vi "readFromXML.vi"(8 "error in (no error)":errorcluster, 10 "XML in":string, 11 "RotOffset in":refnum<class "RotOffset.lvclass">) -> (0 "error out":errorcluster, 3 "RotOffset out":refnum<class "RotOffset.lvclass">)   [LabVIEW 2022 SP3, in "TCSDataDefinitions.lvlib" / "TCSCommand.lvlib" / "OffsetCommands.lvlib" / "RotOffset.lvclass"]
uses:
  RotOffset.lvclass
  <userlib>/Common/UnitsAndXML/FlattenItemWithUnitToXML/FlattenPlaneAngleToXML/PlaneAngleUnit.ctl
  RotOffset.lvclass/RotOffset.ctl
  RotatorOffsetCommands/RotatorOffsetCommands.lvclass
  <userlib>/Common/UnitsAndXML/UnitsAndXML.lvlib
  <userlib>/Common/XML/XMLParser/XMLParser.lvclass
panel:
  out "iaa":dbl[unit]
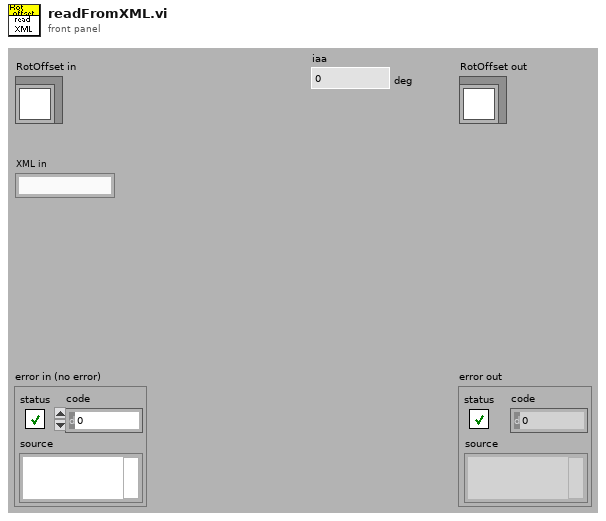
[diagram p1: front panel]
types:
  T1 = typedef "UnitsAndXML.lvlib/PlaneAngleUnit.ctl" = enum16{"rad", "deg", "'", "\""}
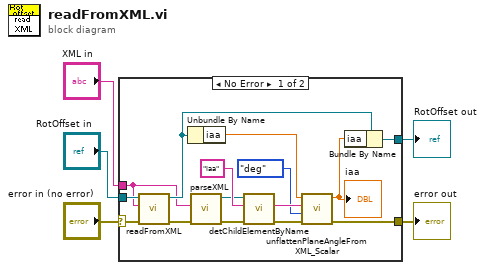
[diagram p0: block diagram]
diagram:
  n1 = case shown="No Error" "error in (no error)" {
    selector: "error in (no error)" -> [w14 w22]
    tunnel: [w8 w22] -> w4
    tunnel: [w18 w21] -> w2
    tunnel: "RotOffset in" -> [w17 w21]
    tunnel: "XML in" -> [w15 _]
    frame No Error {
      n2 = call-parent "readFromXML.vi"("error in (no error)"=w14, "XML in"=w15, "RotatorOffsetCommands in"=w17) -> ("error out"=w13:errorcluster, "RotatorOffsetCommands out"=w16:refnum<class "RotOffset.lvclass">)  [unwired: 7 out]
      n3 = Unbundle By Name(w16) -> ("iaa"=w12:dbl[unit])
      n4 = call <userlib>:"parseXML.vi"("error in (no error)"=w13, "XMLString in"=w15) -> ("error out"=w20:errorcluster, "Element out"=w6:refnum<class "XMLParser.lvclass">)  [unwired: 8 in]
      n5 = call <userlib>:"detChildElementByName.vi"("error in (no error)"=w20, "childName"="iaa" ("ChildName"), "Element in"=w6) -> ("error out"=w10:errorcluster, "childXML"=w11:string)  [unwired: 5 in, 2 out]
      n6 = call <userlib>:"unflattenPlaneAngleFromXML_Scalar.vi"("error in (no error)"=w10, "planeAngleUnitInXML"=PlaneAngleUnit."deg", "xmlString"=w11, "planeAngleForType"=w12) -> ("error out"=w8:errorcluster, "planeAngle"=w7:dbl[unit])  [unwired: 6 in]
      "iaa" <- w7
      n7 = Bundle By Name(cluster=w16, "iaa"=w7) -> (w18:refnum<class "RotOffset.lvclass">)
    }
    frame Error {
    }
  }
  "error out" <- w4
  "RotOffset out" <- w2
